vi "rectangle_to_freehand_line.vi"(8 "Error In":errorcluster, 11 "Input Rect":i32[](array[numeric])) -> (0 "Error Out":errorcluster, 2 "y":i32[](array[numeric]), 3 "x":i32[](array[numeric]))   [LabVIEW 2019]
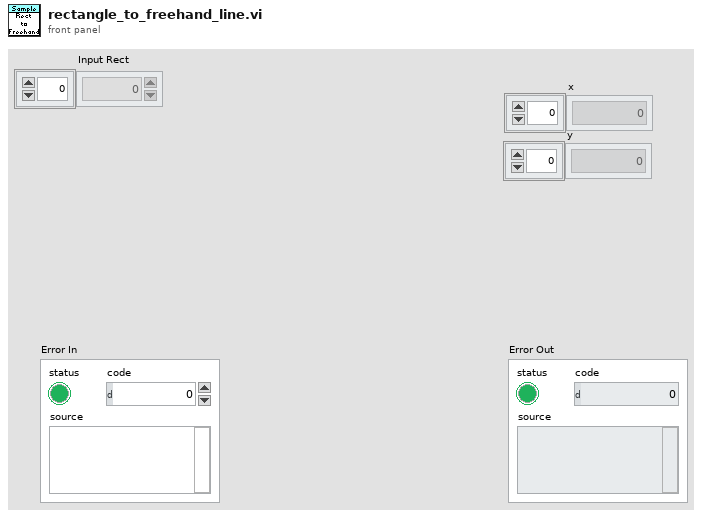
[diagram p1: front panel]
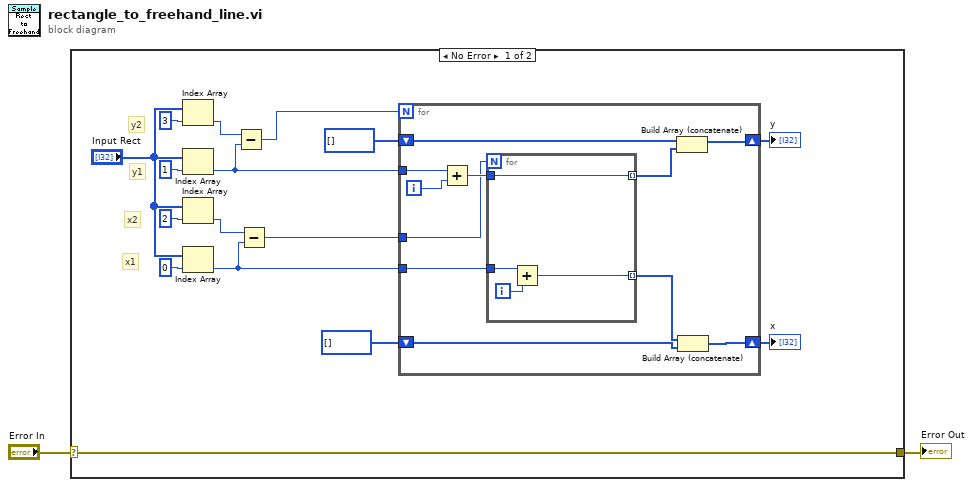
[diagram p0: block diagram]
diagram:
  n1 = case shown="No Error" "Error In" {
    selector: "Error In" -> [w18 w34]
    tunnel: [w18 w34] -> w1
    frame No Error {
      # "y2"
      # "y1"
      # "x2"
      # "x1"
      n2 = Index Array(array="Input Rect", index=3) -> (element=w12:i32)
      n3 = Index Array(array="Input Rect", index=1) -> (element=w9:i32)
      n4 = Index Array(array="Input Rect", index=2) -> (element=w11:i32)
      n5 = Index Array(array="Input Rect", index=0) -> (element=w7:i32)
      n6 = Subtract(x=w12, y=w9) -> (x-y=w10:i32)
      n7 = Subtract(x=w11, y=w7) -> (x-y=w8:i32)
      n8 = for {
        N: w10 -> [_]
        tunnel: w9 -> [w29]
        tunnel: w8 -> [w25]
        tunnel: w7 -> [w27]
        shift-right: [w22] -> w4
        shift-left: i32[] [] -> [w24]
        shift-right: [w21] -> w3
        shift-left: i32[] [] -> [w20]
        i -> [w28]
        n9 = Add(x=w29, y=w28) -> (x+y=w26:i32)
        n10 = for {
          N: w25 -> [_]
          tunnel: w27 -> [w33]
          tunnel: w26 -> [w31]
          tunnel: [w31] -> w23 mode=indexing
          tunnel: [w30] -> w19 mode=indexing
          i -> [w32]
          n11 = Add(x=w33, y=w32) -> (x+y=w30:i32)
        }
        n12 = Build Array (concatenate)(w24, w23) -> (w22:i32[])
        n13 = Build Array (concatenate)(w19, w20) -> (w21:i32[])
      }
      "y" <- w4
      "x" <- w3
    }
    frame Error {
    }
  }
  "Error Out" <- w1
